vi "clear Session Data.vi"(0 "Session in":refnum<class "Process Bar.lvclass">, 11 "error in":errorcluster) -> (4 "Session out":refnum<class "Process Bar.lvclass">, 15 "error out":errorcluster)   [LabVIEW 2018, in "Process Bar.lvclass"]
uses:
  Process Bar.lvclass
  <userlib>/_Session Fwk/Session - Root.lvclass
  C:/Program Files/National Instruments/LabVIEW 2018/user.lib/_Session Fwk/Session - Root.lvclass
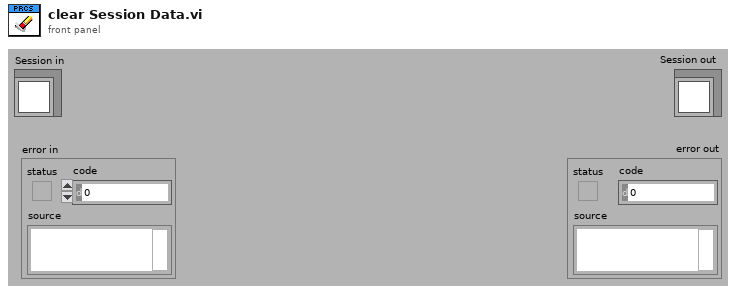
[diagram p1: front panel]
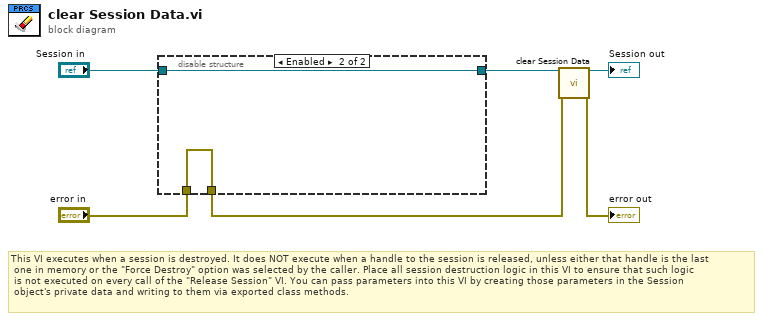
[diagram p0: block diagram]
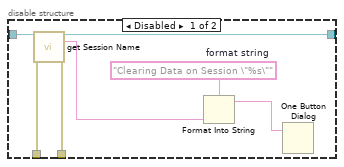
[diagram p2: hidden frame]
diagram:
  # "This VI executes when a session is destroyed. It does NOT execute when a handle to the session is released, unless either that handle is the last\n one in memory or the \"Force Destroy\" option was selected by the caller. Place all session destruction logic in this VI to ensure that such logic\n is not executed on every call of the \"Release Session\" VI. You can pass parameters into this VI by creating those parameters in the Session \n object's private data and writing to them via exported class methods."
  n1 = disable-structure shown="Enabled" {
    disable-tunnel: "Session in" -> [w13 w15]
    disable-tunnel: [w12 w15] -> w5
    disable-tunnel: "error in" -> [w8 w14]
    disable-tunnel: [w7 w14] -> w1
    frame Disabled {
      w11 = "Clearing Data on Session \"%s\""  # format string
      n2 = call <userlib>:"get Session Name.vi"("OBJ - Session in"=w13, "error in (no error)"=w8) -> ("OBJ - Session out"=w12:refnum<class "Process Bar.lvclass">, "Session Name"=w9:string, "error out"=w7:errorcluster)  [unwired: 11 in]
      n3 = Format Into String(format string=w11, w9) -> (resulting string=w10:string)  [unwired: 2 in, 1 out]
      n4 = One Button Dialog(message=w10) -> ()  [unwired: 1 in, 1 out]
    }
    frame Enabled {
    }
  }
  n5 = call-parent "clear Session Data.vi"("OBJ - Measurement Session in"=w5, "error in"=w1) -> ("OBJ - Measurement Session out"=→"Session out":refnum<class "Process Bar.lvclass">, "error out"=→"error out":errorcluster)  [unwired: 12 in]
